vi "Gaussian White Noise PtByPt.vi"(1 "initialize":bool, 2 "seed":i32=-1, 3 "standard deviation":dbl=1.0 format="%0.2f") -> (0 "Gaussian white noise":dbl format="%0.2f")   [LabVIEW 2020, in "NI_PtbyPt.lvlib"]
doc: "Generates a Gaussian-distributed, pseudorandom pattern whose statistical profile is (mu, sigma) = (0, s), where s is <B>standard deviation</B>."
uses:
  NI_PtbyPt.lvlib
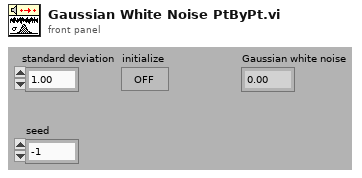
[diagram p1: front panel]
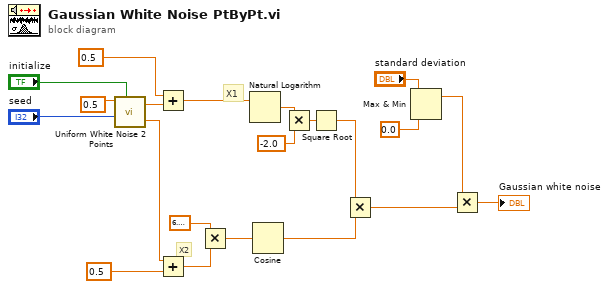
[diagram p0: block diagram]
diagram:
  # "X2"
  # "X1"
  n1 = call "Uniform White Noise 2 Points.vi"("amplitude"=0.5, "seed"="seed", "initialize"="initialize") -> ("uniform white noise 1"=w6:dbl, "uniform white noise 2"=w1:dbl)  [unwired: 2 in]
  n2 = Add(x=0.5, y=w6) -> (x+y=w8:dbl)
  n3 = Add(x=w1, y=0.5) -> (x+y=w10:dbl)
  n4 = Multiply(x=6.283185307179586, y=w10) -> (x*y=w17:dbl)
  n5 = Natural Logarithm(1:w8) -> (0:w21:dbl)
  n6 = Cosine(x=w17) -> (cos(x)=w15:dbl)
  n7 = Multiply(x=w21, y=-2.0) -> (x*y=w19:dbl)
  n8 = Square Root(x=w19) -> (sqrt(x)=w16:dbl)
  n9 = Multiply(x=w16, y=w15) -> (x*y=w9:dbl)
  n10 = Max & Min(x="standard deviation", y=0.0) -> (max(x,y)=w12:dbl)  [unwired: 1 out]
  n11 = Multiply(x=w12, y=w9) -> (x*y=→"Gaussian white noise":dbl)
